vi "24HP_Process.vi"(0 "All samples in":sgl[][](array[numeric]), 1 "24HP Ch No":i16[](array[numeric]), 2 "Analysis info Index":i32[](array[numeric]), 3 "Sampling Rate":dbl, 4 "Probe Number":i32) -> ()   [LabVIEW 2020]
uses:
  <vilib>/Analysis/NI_AALBase.lvlib
  <vilib>/Analysis/baseanly.llb/Mean (DBL).vi
  Sub_vis/Upload Data.ctl
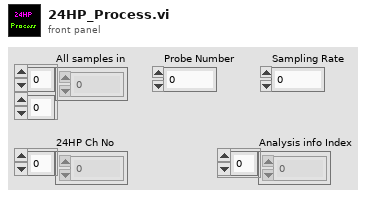
[diagram p1: front panel]
types:
  T1 = typedef "Upload Data.ctl" = enum16{"Voltage Array", "Time Trace Cluster"}
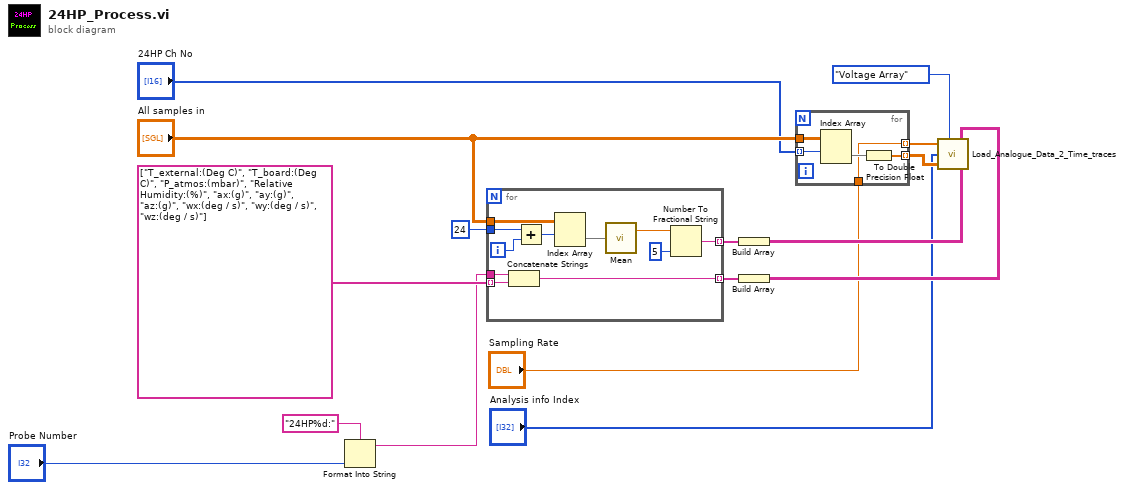
[diagram p0: block diagram]
diagram:
  n1 = Format Into String(format string="24HP%d:", "Probe Number") -> (resulting string=w3:string)  [unwired: 2 in, 1 out]
  n2 = for {
    tunnel: "All samples in" -> [w27]
    tunnel: 24 -> [w25]
    tunnel: w3 -> [w23]
    tunnel: string[] ["T_external:(Deg C)", "T_board:(Deg C)", "P_atmos:(mbar)", "Relative Humidity:(%)", "ax:(g)", "ay:(g)", "az:(g)", "wx:(deg / s)", "wy:(deg / s)", "wz:(deg / s)"] -> [w22] mode=indexing
    tunnel: [w18] -> w12 mode=indexing
    tunnel: [w17] -> w11 mode=indexing
    i -> [w26]
    n3 = Concatenate Strings(w23, w22) -> (w17:string)
    n4 = Add(x=w25, y=w26) -> (x+y=w24:i32)
    n5 = Index Array(array=w27, index (row)=w24) -> (element=w21:sgl[])  [unwired: 1 in]
    n6 = call-poly <vilib>:"Mean.vi"("X"=w21) -> ("mean"=w20:dbl)  [unwired: 1 out]
    n7 = Number To Fractional String(number=w20, precision (6)=i16 5) -> (F-format string=w18:string)  [unwired: 2 in]
  }
  n8 = Build Array(w12) -> (w14:string[][])
  n9 = Build Array(w11) -> (w13:string[][])
  n10 = for {
    tunnel: "24HP Ch No" -> [w31] mode=indexing
    tunnel: "All samples in" -> [w32]
    tunnel: "Sampling Rate" -> [w28]
    tunnel: [w29] -> w7 mode=indexing
    tunnel: [w28] -> w8 mode=indexing
    n11 = Index Array(array=w32, index (row)=w31) -> (element=w30:sgl[])  [unwired: 1 in]
    n12 = To Double Precision Float(number=w30) -> (double precision float=w29:dbl[])
  }
  n13 = call "Load_Analogue_Data_2_Time_traces.vi"("Sampling Rate (Hz)"=w8, "Mode"=Upload_Data."Voltage Array", "Index"="Analysis info Index", "Voltage Array"=w7, "Metadata Names"=w13, "Metadata Values"=w14) -> ()  [unwired: 1 in]
